vi "ProducerConsumerEvents.vi"() -> ()   [LabVIEW 2015]
doc: "Use this template to build a producer/consumer design pattern with events to produce queue items. Use this design pattern instead of the User Interface Event Handler pattern for user interfaces when you want to execute code asynchronously in response to an event without slowing the user interface responsiveness."
uses:
  C:/Program Files (x86)/National Instruments/LabVIEW 2015/examples/Data Communication/Protocols/TCP/TCP Multiple Connections/controls/TCP Multiple Connections State.ctl
  C:/Program Files (x86)/National Instruments/LabVIEW 2015/examples/Data Communication/Protocols/TCP/TCP Multiple Connections/controls/TCP Multiple Connections Data.ctl
panel:
  out "# of Connections":i32
  in  "Stop":bool
  in  "Enqueue Element":bool
  in  "stop":bool
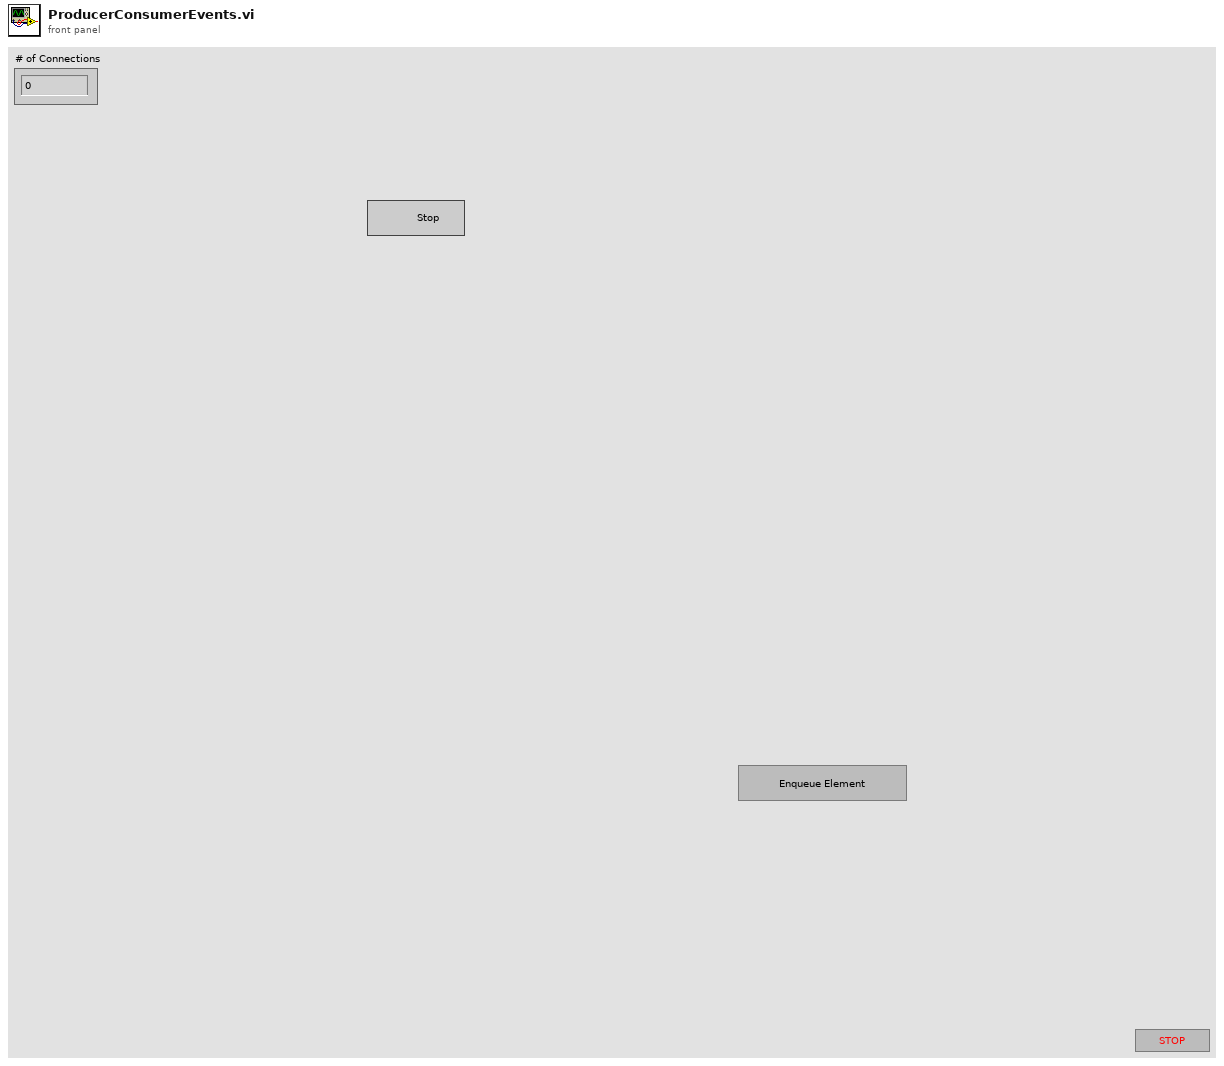
[diagram p1: front panel]
types:
  T1 = typedef "TCP Multiple Connections Data.ctl" = cluster{"Clients":refnum<k5>[], "Listener":refnum<k5>}
  T2 = typedef "TCP Multiple Connections State.ctl" = enum16{"Initialize", "Status Check", "Send Data", "Stop"}
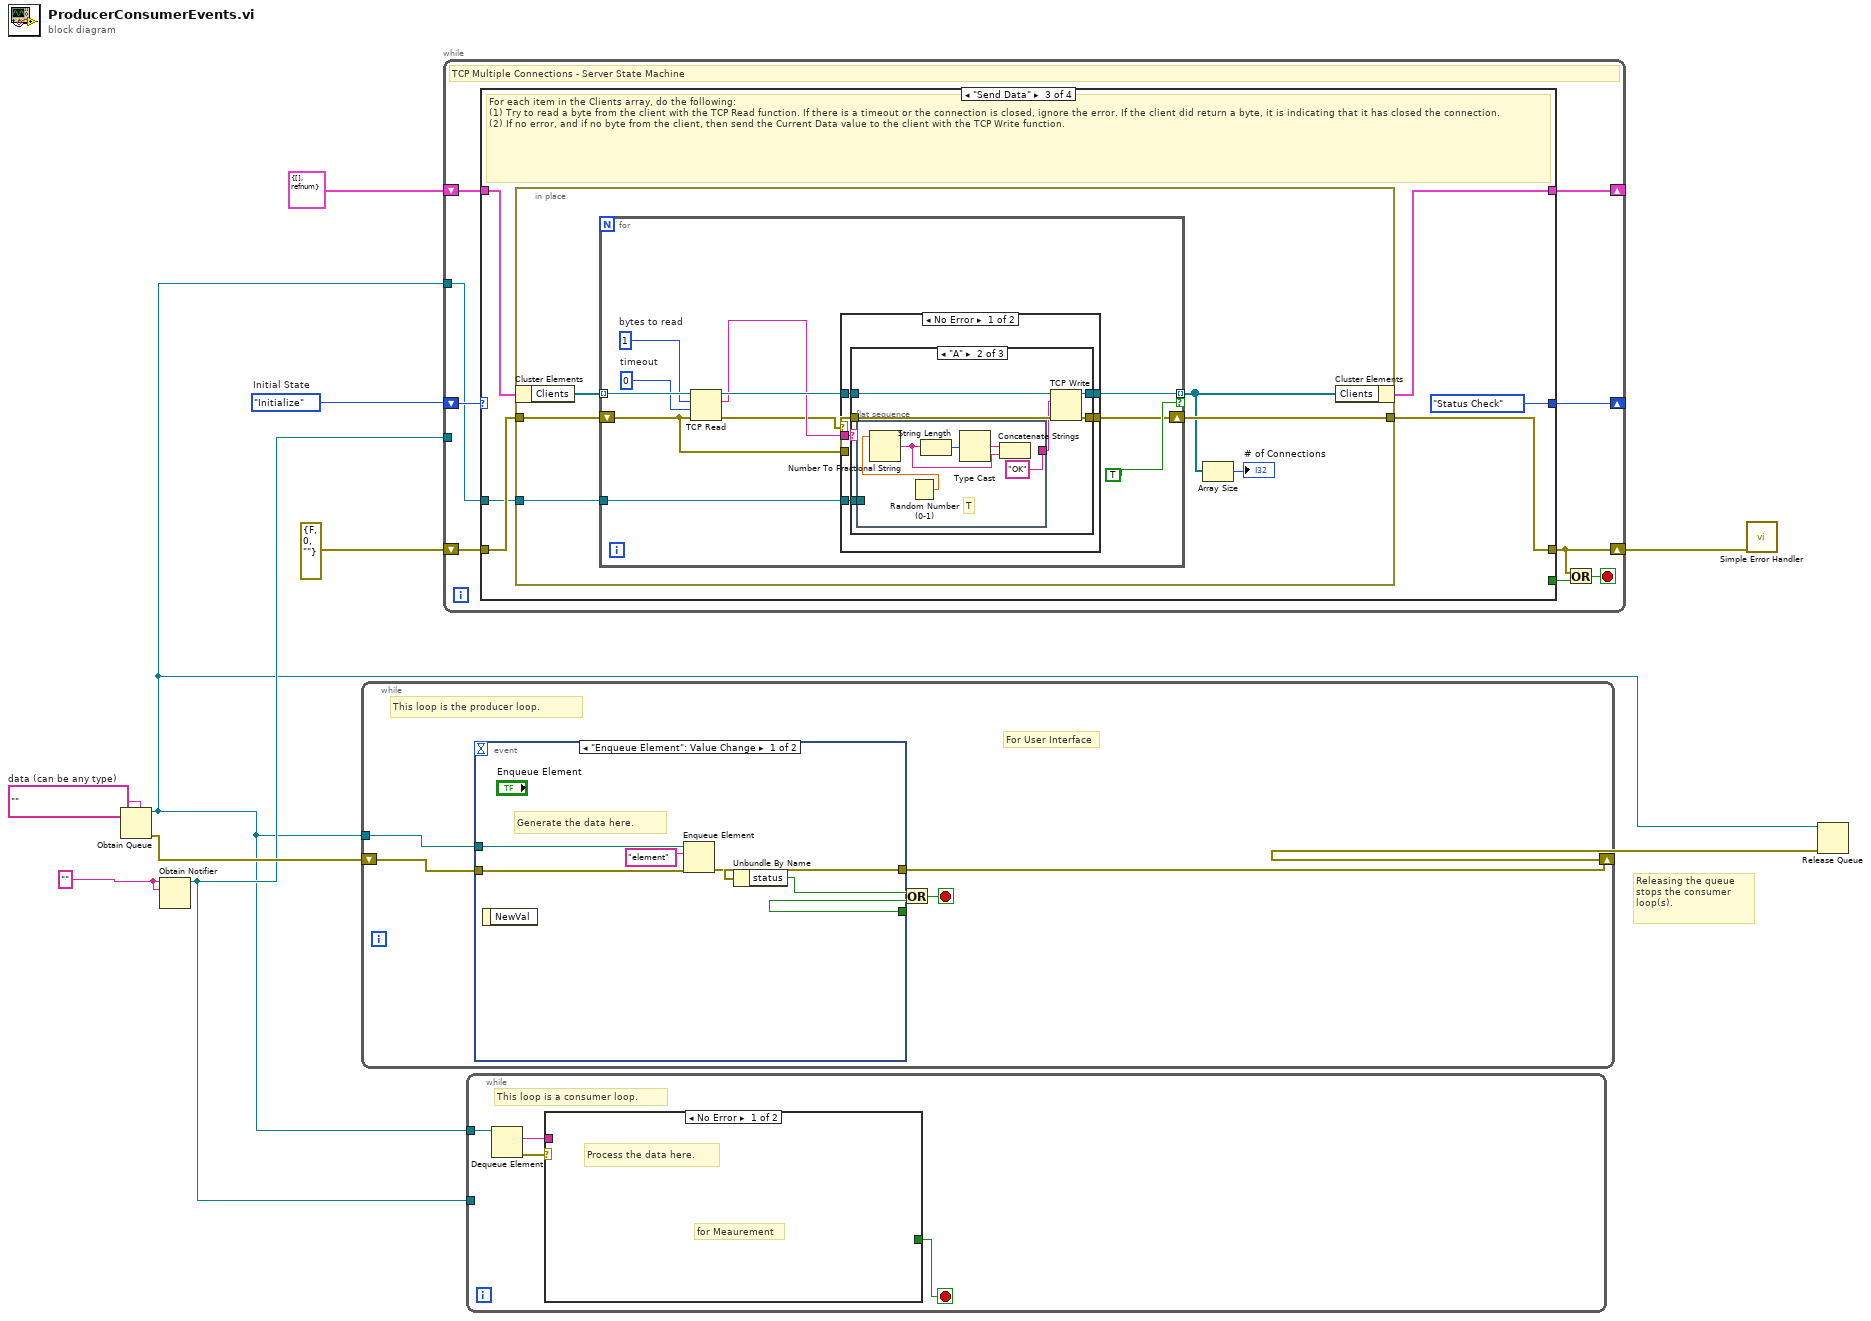
[diagram p0: block diagram]
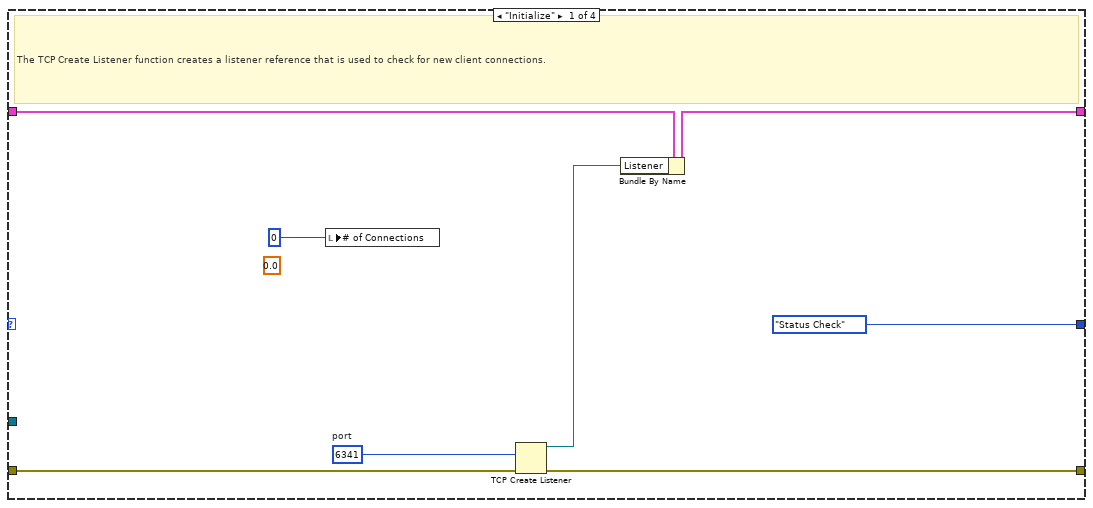
[diagram p2: hidden frame]
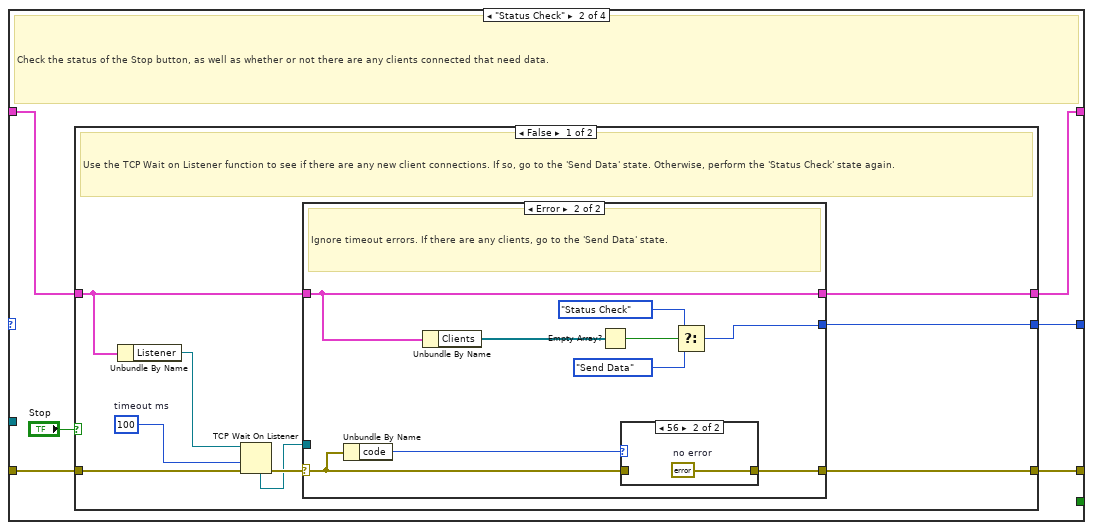
[diagram p3: hidden frame]
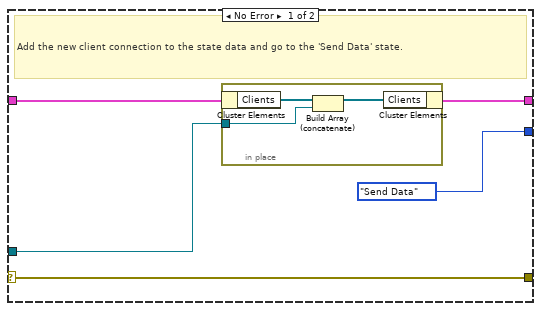
[diagram p4: hidden frame]
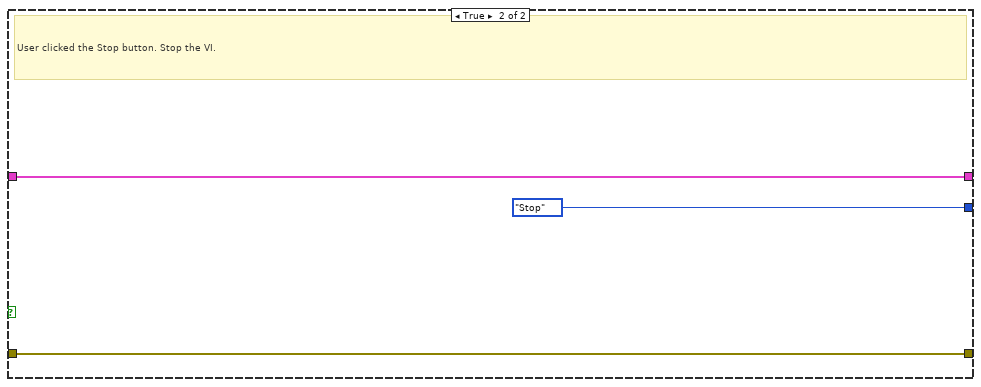
[diagram p6: hidden frame]
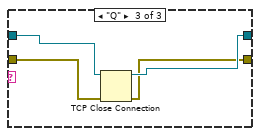
[diagram p8: hidden frame]
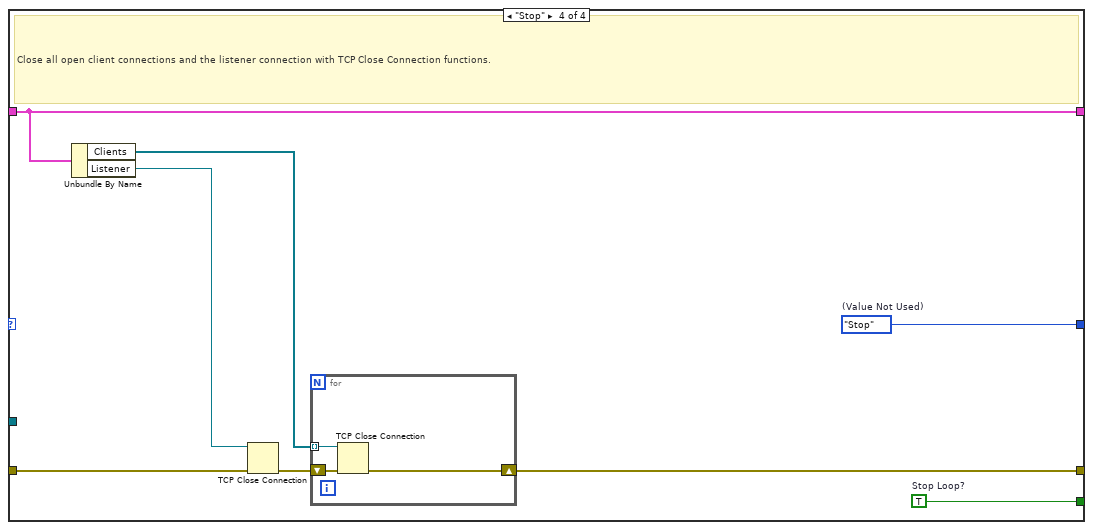
[diagram p10: hidden frame]
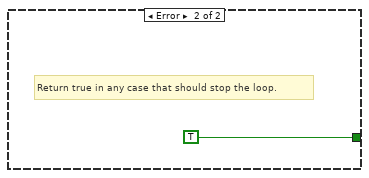
[diagram p11: hidden frame]
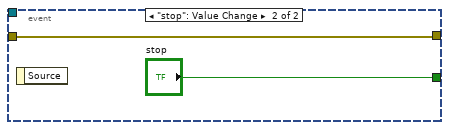
[diagram p12: hidden frame]
diagram:
  w1 = "" ("name (unnamed)")
  w7 = TCP_Multiple_Connections_State."Initialize"  # Initial State
  w8 = ""  # data (can be any type)
  # "Releasing the queue stops the consumer loop(s)."
  n1 = Obtain Queue(element data type=w8) -> (queue out=w2:refnum<queue>, error out=w10:errorcluster)  [unwired: 4 in, 1 out]
  n2 = Obtain Notifier(name (unnamed)=w1, notification data type=w1) -> (notifier out=w3:refnum<notifier>)  [unwired: 2 in, 2 out]
  n3 = while {
    shift-right: [w12] -> w9
    shift-left: w10 -> [w15]
    tunnel: w2 -> [w16]
    stop <- w13 stop-if-true
    # "For User Interface"
    # "This loop is the producer loop."
    n4 = event shown="[0] \"Enqueue Element\": Value Change" {
      selector: _ -> [_ _]
      dyn-events: _ -> [_ _]
      timeout: _ -> [_ _]
      tunnel: w16 -> [w20 _]
      tunnel: w15 -> [w19 w21]
      tunnel: [w18 w21] -> w12
      tunnel: [_ "stop"] -> w14
      event "Enqueue Element": Value Change {
        # "Generate the data here."
        n5 = event-data() -> ()  [unwired: 1 in, 1 out]
        n6 = Enqueue Element(queue=w20, element="element", error in (no error)=w19) -> (error out=w18:errorcluster)  [unwired: 1 in, 2 out]
      }
      event "stop": Value Change {
        n7 = event-data() -> ()  [unwired: 1 in, 1 out]
      }
    }
    n8 = Unbundle By Name(w12) -> ("status"=w11:bool)
    n9 = Or(x=w11, y=w14) -> (x .or. y?=w13:bool)
  }
  n10 = while {
    shift-right: [w30] -> _
    shift-left: w7 -> [w31]
    shift-right: [w28] -> _
    shift-left: T1 {"Clients"=[], "Listener"=refnum} ("Data") -> [w29]
    shift-right: [w24] -> w4
    shift-left: errorcluster {"status"=FALSE, "code"=0, "source"=""} ("error constant") -> [w27]
    tunnel: w2 -> [w23]
    tunnel: w3 -> [_]
    stop <- w25 stop-if-true
    # "TCP Multiple Connections - Server State Machine"
    n11 = case shown="\"Send Data\"" w31 {
      tunnel: [TCP_Multiple_Connections_State."Status Check" ("States") w45 TCP_Multiple_Connections_State."Status Check" ("States") w125] -> w30
      tunnel: [_ _ _ w132] -> w26
      tunnel: w29 -> [w37 w41 w80 w131]
      tunnel: [w36 w40 w79 w131] -> w28
      tunnel: w27 -> [w39 w44 w82 w130]
      tunnel: [w38 w43 w81 w128] -> w24
      tunnel: w23 -> [_ _ w77 _]
      frame "Initialize" {
        (unwired) 0.0 ("Current Data")
        w34 = u16 6341  # port
        # "The TCP Create Listener function creates a listener reference that is used to check for new client connections."
        n12 = local write "# of Connections"(0 ("Number of Client Connections")) -> ()
        n13 = TCP Create Listener(8:w39, 10:w34) -> (0:w38:errorcluster, 3:w35:refnum<k5>)  [unwired: 4 out]
        n14 = Bundle By Name(cluster=w37, "Listener"=w35) -> (w36:T1)
      }
      frame "Status Check" {
        # "Check the status of the Stop button, as well as whether or not there are any clients connected that need data."
        n15 = case shown="False" "Stop" {
          tunnel: [w54 TCP_Multiple_Connections_State."Stop" ("States")] -> w45
          tunnel: w44 -> [w53 w76]
          tunnel: [w46 w76] -> w43
          tunnel: w41 -> [w49 w75]
          tunnel: [w48 w75] -> w40
          frame False {
            w52 = 100  # timeout ms
            # "Use the TCP Wait on Listener function to see if there are any new client connections. If so, go to the 'Send Data' state. Otherwise, perform the 'Status Check' state again."
            n16 = Unbundle By Name(w49) -> ("Listener"=w47:refnum<k5>)
            n17 = TCP Wait On Listener(8:w53, 9:w52, 11:w47) -> (0:w51:errorcluster, 4:w50:refnum<k5>)  [unwired: 4 out]
            n18 = case shown="Error" w51 {
              selector: w51 -> [w57 w71]
              tunnel: [TCP_Multiple_Connections_State."Send Data" ("States") w65] -> w54
              tunnel: w50 -> [w58 _]
              tunnel: w49 -> [w59 w68]
              tunnel: [w56 w68] -> w48
              tunnel: [w57 w69] -> w46
              frame No Error {
                # "Add the new client connection to the state data and go to the 'Send Data' state."
                n19 = in-place {
                  in-place-border: w58 -> [w60]
                  n20 = in-place-cluster #1(w59) -> ("Clients"=w62:refnum<k5>[])
                  n21 = Build Array (concatenate)(w62, w60) -> (w61:refnum<k5>[])
                  n22 = in-place-cluster #1("Clients"=w61) -> (w56:T1)
                }
              }
              frame Error {
                # "Ignore timeout errors. If there are any clients, go to the 'Send Data' state."
                n23 = Unbundle By Name(w71) -> ("code"=w70:i32)
                n24 = Unbundle By Name(w68) -> ("Clients"=w67:refnum<k5>[])
                n25 = Empty Array?(array=w67) -> (empty?=w66:bool)
                n26 = case shown="56" w70 {
                  tunnel: w71 -> [w72 _]
                  tunnel: [w72 w73] -> w69
                  frame Default {
                  }
                  frame 56 {
                    w73 = errorcluster {"status"=FALSE, "code"=0, "source"=""}  # no error
                  }
                }
                n27 = Select(t=TCP_Multiple_Connections_State."Status Check" ("States"), s=w66, f=TCP_Multiple_Connections_State."Send Data" ("States")) -> (s? t:f=w65:T2)
              }
            }
          }
          frame True {
            # "User clicked the Stop button. Stop the VI."
          }
        }
      }
      frame "Send Data" {
        # "For each item in the Clients array, do the following:\n(1) Try to read a byte from the client with the TCP Read function. If there is a timeout or the connection is closed, ignore the error. If the client did return a byte, it is indicating that it has closed the connection.\n(2) If no error, and if no byte from the client, then send the Current Data value to the client with the TCP Write function."
        n28 = in-place {
          in-place-border: w82 -> [w88]
          in-place-border: [w87] -> w81
          in-place-border: w77 -> [w83]
          n29 = in-place-cluster #2(w80) -> ("Clients"=w85:refnum<k5>[])
          n30 = for {
            tunnel: w85 -> [w99] mode=indexing
            shift-right: [w92] -> w87
            shift-left: w88 -> [w91]
            tunnel: [w94] -> w84 mode=indexing if=TRUE
            tunnel: w83 -> [w90]
            w96 = 0  # timeout
            w97 = 1  # bytes to read
            n31 = TCP Read(connection ID=w99, bytes to read=w97, error in (no error)=w91, 9:w96) -> (connection ID out=w98:refnum<k5>, data out=w95:string, error out=w89:errorcluster)  [unwired: 1 out]
            n32 = case shown="No Error" w89 {
              tunnel: w98 -> [w105 w124]
              tunnel: w95 -> [w104 _]
              tunnel: [w103 w124] -> w94
              tunnel: [w102 w123] -> w92
              tunnel: w91 -> [w101 w123]
              tunnel: w90 -> [w100 _]
              frame No Error {
                n33 = case shown="\"A\"" w104 {
                  tunnel: [w106 w113 w120] -> w102
                  tunnel: w105 -> [w107 w112 w122]
                  tunnel: [w107 w111 w121] -> w103
                  tunnel: w101 -> [w106 w110 w119]
                  tunnel: w100 -> [_ w109 _]
                  frame "False", Default {
                  }
                  frame "A" {
                    n34 = flat-sequence {
                      tunnel: ["OK"] -> w108
                      tunnel: w109 -> [_]
                      frame #0 {
                        # "T"
                        n35 = Random Number (0-1)() -> (number: 0 to 1=w118:dbl)
                        n36 = Number To Fractional String(number=w118) -> (F-format string=w115:string)  [unwired: 3 in]
                        n37 = String Length(string=w115) -> (length=w116:i32)
                        n38 = Type Cast(x=w116) -> (*(type *) &x=w117:string)  [unwired: 1 in]
                        n39 = Concatenate Strings(w117, w115) -> ()  [unwired: 1 out]
                      }
                    }
                    n40 = TCP Write(connection ID=w112, data in=w108, error in (no error)=w110) -> (connection ID out=w111:refnum<k5>, error out=w113:errorcluster)  [unwired: 2 out]
                  }
                  frame "Q" {
                    n41 = TCP Close Connection(connection ID=w122, error in (no error)=w119) -> (connection ID out=w121:refnum<k5>, error out=w120:errorcluster)  [unwired: 1 out]
                  }
                }
              }
              frame Error {
              }
            }
          }
          n42 = Array Size(array=w84) -> (size(s)=→"# of Connections":i32)
          n43 = in-place-cluster #2("Clients"=w84) -> (w79:T1)
        }
      }
      frame "Stop" {
        w125 = TCP_Multiple_Connections_State."Stop"  # (Value Not Used)
        w132 = TRUE  # Stop Loop?
        # "Close all open client connections and the listener connection with TCP Close Connection functions."
        n44 = Unbundle By Name(w131) -> ("Clients"=w129:refnum<k5>[], "Listener"=w126:refnum<k5>)
        n45 = TCP Close Connection(connection ID=w126, error in (no error)=w130) -> (error out=w127:errorcluster)  [unwired: 1 in, 1 out]
        n46 = for {
          shift-right: [w134] -> w128
          shift-left: w127 -> [w135]
          tunnel: w129 -> [w133] mode=indexing
          n47 = TCP Close Connection(connection ID=w133, error in (no error)=w135) -> (error out=w134:errorcluster)  [unwired: 1 in, 1 out]
        }
      }
    }
    n48 = Or(x=w24, y=w26) -> (x .or. y?=w25:bool)
  }
  n49 = while {
    tunnel: w2 -> [w139]
    tunnel: w3 -> [_]
    stop <- w136 stop-if-true
    # "This loop is a consumer loop."
    n50 = Dequeue Element(queue=w139) -> (element=w137:string, error out=w138:errorcluster)  [unwired: 2 in, 2 out]
    n51 = case shown="No Error" w138 {
      tunnel: w137 -> [_ _]
      tunnel: [_ TRUE] -> w136
      frame No Error {
        # "for Meaurement"
        # "Process the data here."
      }
      frame Error {
        # "Return true in any case that should stop the loop."
      }
    }
  }
  n52 = call <vilib>:"Simple Error Handler.vi"("error in (no error)"=w4) -> ()  [unwired: 4 in, 5 out]
  n53 = Release Queue(queue=w2, error in (no error)=w9) -> ()  [unwired: 1 in, 3 out]
